vi "receive.vi"() -> ()   [LabVIEW 2017]
uses:
  <vilib>/Instr/_visa.llb/VISA Configure Serial Port (Instr).vi
panel:
  in  "baud rate":u32(ring)=9600 caption="波特率" items=["9600"=9600]
  out "Y":sgl
  out "X":sgl
  out "XY Graph":cluster{"Y":dbl[], "Y":dbl[]}[](graph) caption="XY图"
  in  "?":bool
  in  "VISA resource name":refnum<visa-resource-name> caption="串口源"
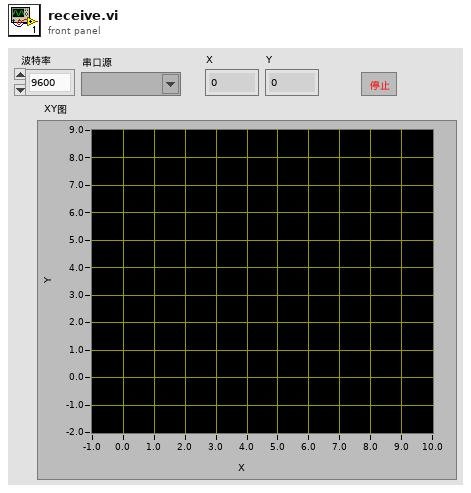
[diagram p1: front panel]
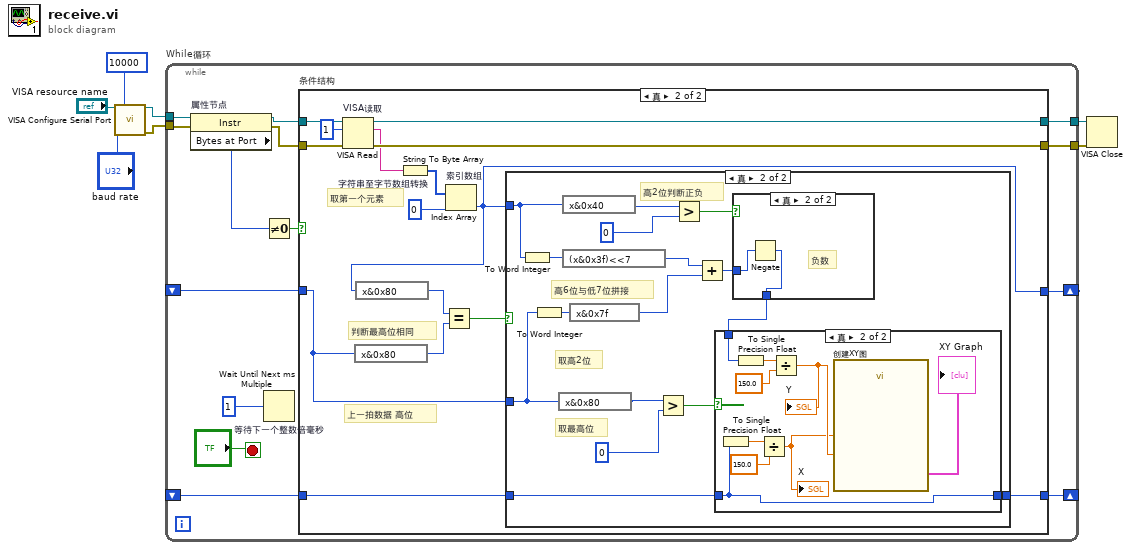
[diagram p0: block diagram]
diagram:
  n1 = call-poly "VISA Configure Serial Port"("VISA resource name"="VISA resource name", "timeout (10sec)"=u32 10000, "baud rate (9600)"="baud rate") -> ("VISA resource name out"=w5:refnum<visa-resource-name>, "error out"=w4:errorcluster)  [unwired: 11 in]
  n2 = while "While循环" {
    tunnel: w5 -> [w20]
    tunnel: [w15] -> w3
    tunnel: w4 -> [w19]
    tunnel: [w14] -> w2
    shift-right: [w12] -> _
    shift-left: _ -> [w11]
    shift-right: [w10] -> _
    shift-left: _ -> [w9]
    stop <- "?" stop-if-true
    n3 = property on="属性节点" class="Instr"(reference=w20, error in=w19) -> (reference out=w18:refnum<visa-resource-name>, error out=w17:errorcluster, "Bytes at Port"=w8:u32)
    n4 = Not Equal To 0?(x=w8) -> (x != 0?=w16:bool)
    n5 = Wait Until Next ms Multiple "等待下一个整数倍毫秒"(millisecond multiple=u32 1 ("毫秒倍数")) -> ()  [unwired: 1 out]
    n6 = case "条件结构" shown="真" w16 {
      tunnel: w18 -> [w25 w40]
      tunnel: w17 -> [w24 w39]
      tunnel: [w25 w38] -> w15
      tunnel: [w24 w37] -> w14
      tunnel: [w23 w31] -> w12
      tunnel: w11 -> [w23 w26]
      tunnel: [w22 w30] -> w10
      tunnel: w9 -> [w22 w29]
      frame False {
      }
      frame True {
        # "上一拍数据 高位"
        # "判断最高位相同"
        # "取第一个元素"
        n7 = VISA Read "VISA读取"(VISA resource name=w40, byte count=u32 1 ("字节总数"), error in (no error)=w39) -> (VISA resource name out=w38:refnum<visa-resource-name>, read buffer=w36:string, error out=w37:errorcluster)  [unwired: 1 out]
        n8 = expression code="x&0x80"(w26) -> (w33:u8)
        n9 = String To Byte Array "字符串至字节数组转换"(string=w36) -> (unsigned byte array=w35:u8[])
        n10 = Index Array "索引数组"(array=w35, index=0) -> (element=w31:u8)
        n11 = expression code="x&0x80"(w31) -> (w34:u8)
        n12 = Equal?(x=w34, y=w33) -> (x = y?=w32:bool)
        n13 = case shown="真" w32 {
          tunnel: w31 -> [_ w42]
          tunnel: w26 -> [_ w49]
          tunnel: [w41 w45] -> w30
          tunnel: w29 -> [w41 w43]
          frame False {
          }
          frame True {
            # "高2位判断正负"
            # "取最高位"
            # "取高2位"
            # "高6位与低7位拼接"
            n14 = To Word Integer(number=w42) -> (16bit integer=w56:i16)
            n15 = To Word Integer(number=w49) -> (16bit integer=w54:i16)
            n16 = expression code="x&0x80"(w49) -> (w47:u8)
            n17 = expression code="x&0x40"(w42) -> (w53:u8)
            n18 = expression code="(x&0x3f)<<7"(w56) -> (w57:i16)
            n19 = expression code="x&0x7f"(w54) -> (w55:i16)
            n20 = Greater?(x=w47, y=u8 0) -> (0:w46:bool)
            n21 = Greater?(x=w53, y=u8 0) -> (0:w51:bool)
            n22 = Add(x=w57, y=w55) -> (x+y=w50:i16)
            n23 = case shown="真" w51 {
              tunnel: w50 -> [w68 w69]
              tunnel: [w68 w70] -> w44
              frame False {
              }
              frame True {
                # "负数"
                n24 = Negate(x=w69) -> (-x=w70:i16)
              }
            }
            n25 = case shown="真" w46 {
              tunnel: [w58 w62] -> w45
              tunnel: w44 -> [w58 w66]
              tunnel: w43 -> [_ w62]
              frame False {
                # "x轴，把x送入下一次循环"
              }
              frame True {
                n26 = To Single Precision Float(number=w62) -> (single precision float=w61:sgl)
                n27 = To Single Precision Float(number=w66) -> (single precision float=w65:sgl)
                n28 = Divide(x=w61, y=sgl 150.0) -> (x/y=w59:sgl)
                "X" <- w59
                n29 = Divide(x=w65, y=sgl 150.0) -> (x/y=w63:sgl)
                "Y" <- w63
                n30 = call "创建XY图"("Y Input"=w63, "X Input"=w59) -> ("XY Graph"=→"XY Graph":cluster{"X":dbl[], "Y":dbl[]}[])  [unwired: 8 in, 1 out]
              }
            }
          }
        }
      }
    }
  }
  n31 = VISA Close(VISA resource name=w3, error in (no error)=w2) -> ()  [unwired: 1 out]
